vi "ge_PwrSpecMag.vi"(4 "dB On (T)":bool=TRUE, 5 "power spectra [dB EU]":cluster{"f0":dbl, "df":dbl, "magnitude":dbl[]}[](array[cluster])) -> (2 "power spectra [dB EU]":cluster{"f0":dbl, "df":dbl, "magnitude":dbl[]}[](array[cluster]))   [LabVIEW 2018]
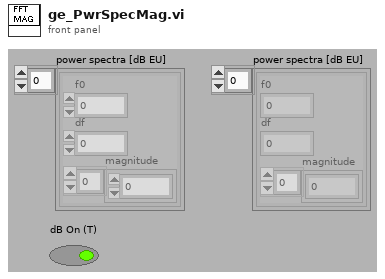
[diagram p1: front panel]
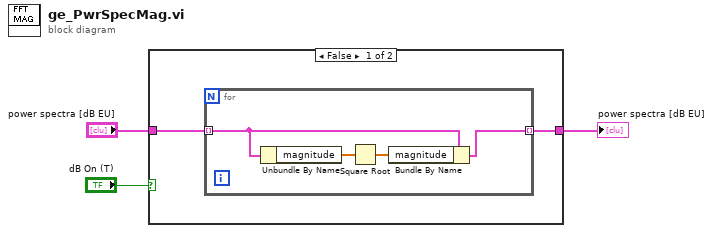
[diagram p0: block diagram]
diagram:
  n1 = case shown="False" "dB On (T)" {
    tunnel: "power spectra [dB EU]" -> [w5 w10]
    tunnel: [w4 w10] -> w1
    frame False {
      n2 = for {
        tunnel: w5 -> [w9] mode=indexing
        tunnel: [w6] -> w4 mode=indexing
        n3 = Unbundle By Name(w9) -> ("magnitude"=w8:dbl[])
        n4 = Square Root(x=w8) -> (sqrt(x)=w7:dbl[])
        n5 = Bundle By Name(cluster=w9, "magnitude"=w7) -> (w6:cluster{"f0":dbl, "df":dbl, "magnitude":dbl[]})
      }
    }
    frame True {
    }
  }
  "power spectra [dB EU]" <- w1
